vi "Robot Global Data.vi"() -> ()   [LabVIEW 2018]
doc: "This global VI can contain as many global variables as you need. Place a control on the panel, give it a good name. To read or write to it from a VI, drag the icon to the diagram of that VI. You can also drag from the project. Click on the node to change which global you access. You shouldn't have multiple locations writing to a global or it will cause a race-condition."
uses:
  <vilib>/Rock Robotics/WPI/Camera/WPI_CameraImageSize.ctl
  <vilib>/Rock Robotics/WPI/DriverStation/WPI_DriverStationRobotMode2.ctl
panel:
  out "D Brake":dbl
  out "D Time":dbl
  out "D Speed":dbl
  out "Joy 1 Button 9":bool
  out "Joy 1 Button 8":bool
  out "Joy 0 Button 9":bool
  out "Joy 0 Button 8":bool
  out "Lift Speed":dbl
  out "Speed Boost":dbl
  out "Turtle Speed":dbl
  out "Desired Speed":dbl
  out "Rabbit Speed":dbl
  out "Auto Time 2":dbl
  out "Auto Speed 2":dbl
  out "Min Speed":dbl
  out "Drive Speed":dbl
  out "Drift Angle":dbl
  out "Trim Right":dbl
  out "Trim Left":dbl
  out "Auto Time":dbl
  out "Auto Speed":dbl
  out "FMS String":string
  out "Gyro Reset":bool
  out "Joy 1 Button 7":bool
  out "Joy 1 Button 6":bool
  out "Joy 1 Button 5":bool
  out "Joy 1 Button 4":bool
  out "Joy 1 Button 3":bool
  out "Joy 1 Button 2":bool
  out "Joy 1 Button 1":bool
  out "Joy 1 Button 0":bool
  out "Joy 0 Button 7":bool
  out "Joy 0 Button 6":bool
  out "Joy 0 Button 5":bool
  out "Joy 0 Button 4":bool
  out "Joy 0 Button 3":bool
  out "Joy 0 Button 2":bool
  out "Joy 0 Button 1":bool
  out "Joy 0 Button 0":bool
  out "Joy 1 Right Y":dbl
  out "Joy 1 Left Y":dbl
  out "Joy 0 Right Y":dbl
  out "Joy 0 Left Y":dbl
  out "Starting Position":dbl
  out "Alliance":dbl
  out "Scale":string
  out "Switch 2":string
  out "Switch 1":string
  out "Drift":dbl
  out "Gyro Rate":dbl
  out "Gyro Raw":dbl
  out "Gyro Value":dbl
  in  "Robot Mode":T1
  in  "image size":T2=enum."320x240"
  in  "Enable Vision":bool
  # "FMS Game Data"
  # "Gyro Data"
  # "Joystick 0 Data"
  # "Joystick 1 Data"
  # "Blue"
  # "Blue"
  # "Green"
  # "Green"
  # "Red"
  # "Red"
  # "Dashboard Control Inputs"
  # "Orange"
  # "Orange"
  # "Left Upper"
  # "Left Upper"
  # "Right Upper"
  # "Right Upper"
  # "Left Trigger"
  # "Left Trigger"
  # "Right Trigger"
  # "Right Trigger"
  # "Select"
  # "Select"
  # "Start"
  # "Start"
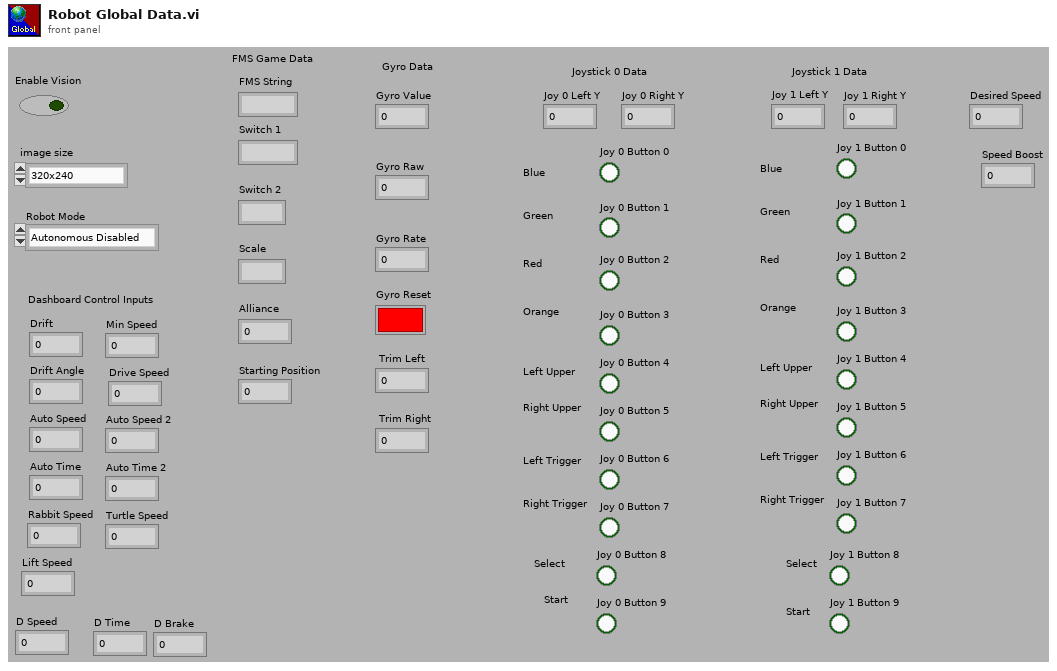
[diagram p1: front panel]
types:
  T1 = typedef "WPI_DriverStationRobotMode2.ctl" = enum16{"Autonomous Disabled", "Autonomous Enabled", "Teleop Disabled", "Teleop Enabled", "Disconnected", "Finish", "Test Disabled", "Test Enabled", "Emergency Stopped"}
  T2 = typedef "WPI_CameraImageSize.ctl" = enum16{"640x480", "320x240", "160x120", "Custom"}
diagram:
